vi "Waveform Generator.vi"(9 "Waveform Parameters":T1 {"Shape" items=["Sine", "Cosine", "DC Level", "Square", "User-Defined"]}, 10 "Digitizing Parameters":T2) -> (2 "Waveform Output":cluster{"Time":dbl[], "Displacement":dbl[]})   [LabVIEW 2014]
doc: "This VI is a waveform generator that can output sin, cos, DC level, square, and misc. defined waveforms. It is able to be used as a sub-VI, along with various customizable input parameters."
uses:
  <vilib>/imath/engines/lvmath2/RunTimeEngine/Managers/WorkSpace/UID Generator.vi
  <vilib>/imath/engines/lvmath2/RunTimeEngine/RunTimeType/NIMS_RunTimeType_From StrictType (excl LVString).vi
  <instcachedir>/0/NIMS_RunTimeType_From StrictType (excl LVString)_15A5391EEA9C4AACB9955AC755B83D29.lvgen/NIMS_RunTimeType_From StrictType (excl LVString)_15A5391EEA9C4AACB9955AC755B83D29_000.vi
  <vilib>/imath/engines/lvmath2/RunTimeEngine/LocalVariableDefStatement/MC_LocalVariableDefStatement_Display.vi
  <vilib>/imath/engines/lvmath2/RunTimeEngine/RangeToken/NIMS_Range.vi
  <instcachedir>/0/NIMS_Range_9BCE657718DF4976A877346C61F22738.lvgen/NIMS_Range_9BCE657718DF4976A877346C61F22738_000.vi
  <vilib>/imathl/engines/lvmath/Functions/Error Handling/Create Error.vi
  <vilib>/imath/engines/lvmath2/RunTimeEngine/ArithmeticOperatorToken/NIMS_ArithmeticOperator_plus.vi
  <instcachedir>/0/NIMS_ArithmeticOperator_plus_48D6EAACA5D645B09F7EC9C016C2DEA8.lvgen/NIMS_ArithmeticOperator_plus_48D6EAACA5D645B09F7EC9C016C2DEA8_004.vi
  <vilib>/imath/engines/lvmath2/RunTimeEngine/BuiltInFunctions/gensignal/NIMS_gensignal(str,RS,RS,RS).vi
  <vilib>/imath/engines/lvmath2/RunTimeEngine/BuiltInFunctions/transpose/NIMS_transpose(GV).vi
  <instcachedir>/0/NIMS_transpose(GV)_1D76875BF542458FA31D2D0CC3E998C0.lvgen/NIMS_transpose(GV)_1D76875BF542458FA31D2D0CC3E998C0_000.vi
  <vilib>/imath/engines/lvmath2/RunTimeEngine/BuiltInFunctions/linramp/NIMS_linramp.vi
  <vilib>/imath/engines/lvmath2/RunTimeEngine/VariableToken/NIMS_VariableToken_CondDefined.vi
  <instcachedir>/0/NIMS_VariableToken_CondDefined_EE8DD211A89249938CE6537267F5C9B3.lvgen/NIMS_VariableToken_CondDefined_EE8DD211A89249938CE6537267F5C9B3_003.vi
  <vilib>/imath/engines/lvmath/Functions/Error Handling/MergeErrorsWrapper.vi
  <vilib>/imath/engines/lvmath2/RunTimeEngine/Managers/SymbolTable/Clear UID.vi
  <vilib>/imath/engines/lvmath2/RunTimeEngine/NodeEndStatement/NIMS_NodeEndStatement_Output.vi
  <instcachedir>/0/NIMS_NodeEndStatement_Output_53EC0D466D134D7ABD903AC30B43404B.lvgen/NIMS_NodeEndStatement_Output_53EC0D466D134D7ABD903AC30B43404B_005.vi
  <vilib>/imath/engines/lvmath2/RunTimeEngine/ErrorHandling/NIMS_Finalize Error.vi
  <vilib>/imath/engines/lvmath2/RunTimeEngine/Managers/SymbolTable/NIMS_WorkSpace.lvlib
panel:
  out "XY Graph":cluster{"t":dbl[], "x":dbl[]}(graph)
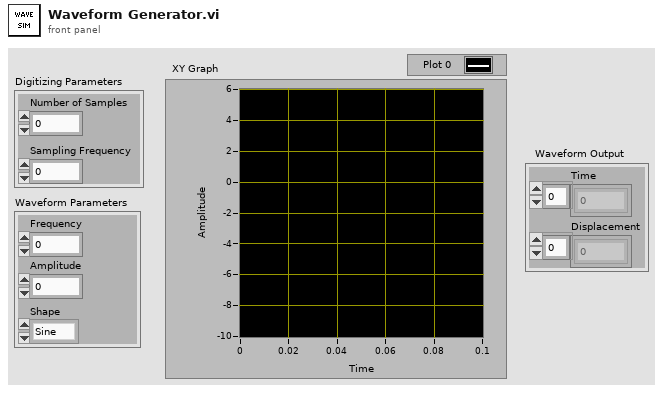
[diagram p1: front panel]
types:
  T1 = cluster{"Frequency ":dbl, "Amplitude ":dbl, "Shape":u16}
  T2 = cluster{"Number of Samples":dbl, "Sampling Frequency":dbl}
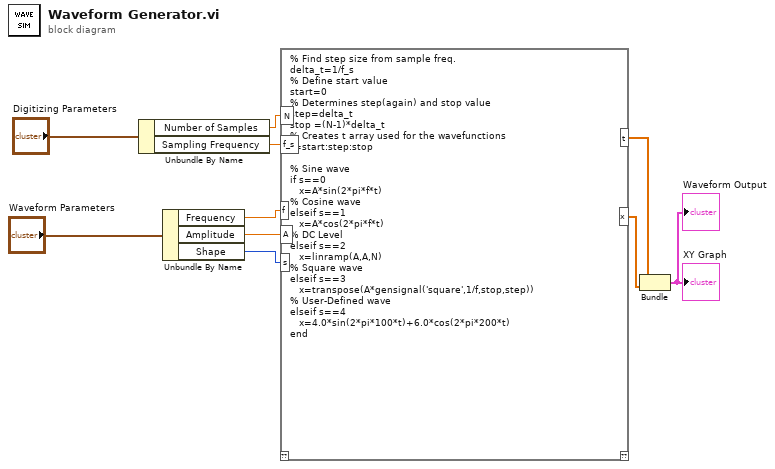
[diagram p0: block diagram]
diagram:
  n1 = Unbundle By Name("Digitizing Parameters") -> ("Number of Samples"=w8:dbl, "Sampling Frequency"=w7:dbl)
  n2 = Unbundle By Name("Waveform Parameters") -> ("Frequency"=w6:dbl, "Amplitude"=w5:dbl, "Shape"=w4:u16)
  n3 = mathscript code="% Find step size from sample freq.\ndelta_t=1/f_s\n% Define start value\nstart=0\n% Determines step(again) and stop value\nstep=delta_t\nstop =(N-1)*delta_t\n% Creates t array used for the wavefunctions\nt=start:step:stop\n\n% Sine wave\nif s==0\n   x=A*sin(2*pi*f*t)\n% Cosine wave\nelseif s==1\n   x=A*cos(2*pi*f*t)\n% DC Level\nelseif s==2\n   x=linramp(A,A,N)\n% Square wave\nelseif s==3\n   x=transpose(A*gensignal('square',1/f,stop,step))\n% User-Defined wave\nelseif s==4\n   x=4.0*sin(2*pi*100*t)+6.0*cos(2*pi*200*t)\nend"("N"=w8, "f_s"=w7, "f"=w6, "A"=w5, "s"=w4) -> ("t"=w3:dbl[], "x"=w2:dbl[])  [unwired: 1 in, 1 out]
  n4 = Bundle("t"=w3, "x"=w2) -> (→"XY Graph" →"Waveform Output":cluster{"t":dbl[], "x":dbl[]})  [unwired: 1 in]
